vi "CoordinateConvert_CartesianToArm.vi"(2 "Y (in)":dbl, 3 "X (in)":dbl) -> (0 "Radius (in)":dbl, 1 "Angle (rad)":dbl)   [LabVIEW 2017]
uses:
  a1a48cbf-37a2-4001-9d38-1b405d9837cb.vi
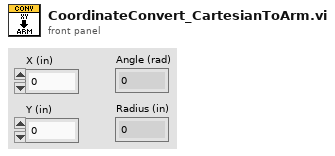
[diagram p1: front panel]
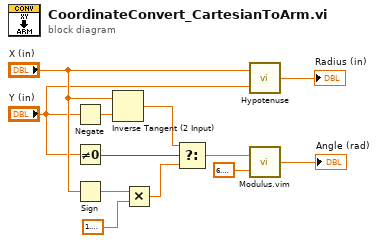
[diagram p0: block diagram]
diagram:
  n1 = Negate(x="Y (in)") -> (-x=w8:dbl)
  n2 = Not Equal To 0?(x="Y (in)") -> (x != 0?=w12:bool)
  n3 = Sign(1:"X (in)") -> (0:w11:dbl)
  n4 = Inverse Tangent (2 Input)(1:w8, 2:"X (in)") -> (0:w7:dbl)
  n5 = Multiply(x=w11, y=1.5707963267948966) -> (x*y=w9:dbl)
  n6 = Select(t=w7, s=w12, f=w9) -> (s? t:f=w6:dbl)
  n7 = call "Hypotenuse.vi"("Y"="Y (in)", "X"="X (in)") -> ("Hypotenuse"=→"Radius (in)":dbl)
  n8 = call "Modulus.vim"("y"=6.283185307179586, "x"=w6) -> ("x%y"=→"Angle (rad)":dbl)
